vi "Destruction.vi"(8 "error in (no error)":errorcluster, 11 "SEQ I64 in":refnum<class "SEQ I64.lvclass">) -> (0 "error out":errorcluster, 3 "SEQ I64 out":refnum<class "SEQ I64.lvclass">)   [LabVIEW 2024, in "SEQ I64.lvclass"]
uses:
  SEQ I64.lvclass
  SEQ I64.lvclass/SEQ I64.ctl
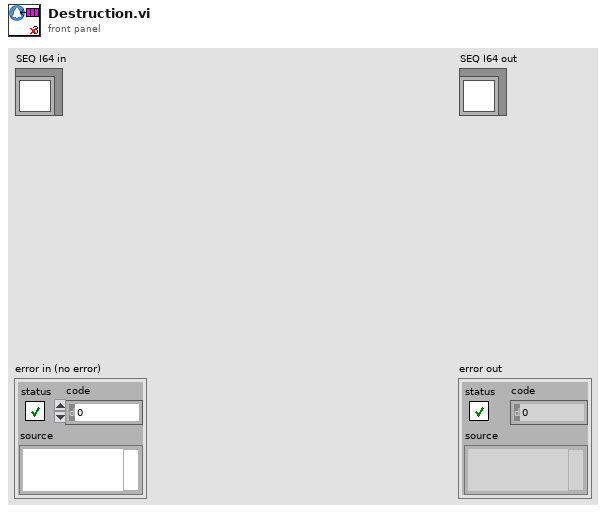
[diagram p1: front panel]
types:
  T1 = typedef "Control 2.ctl" = refnum<queue>
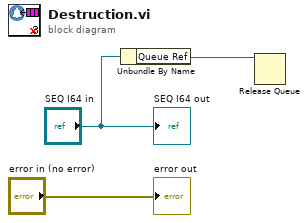
[diagram p0: block diagram]
diagram:
  n1 = Unbundle By Name("SEQ I64 in") -> ("Queue Ref"=w1:T1)
  n2 = Release Queue(queue=w1) -> ()  [unwired: 2 in, 3 out]
  "error out" <- "error in (no error)"
  "SEQ I64 out" <- "SEQ I64 in"
